vi "Status ProgramSetting.vi"(8 "error in (no error)":errorcluster, 10 "Address (0)":i32, 11 "VISA resource name":refnum<visa-resource-name>) -> (0 "error out":errorcluster, 1 "PRGM Name":string, 2 "PRGM area":i32, 3 "VISA resource name out":refnum<visa-resource-name>, 5 "End condition":T1)   [LabVIEW 2021, in "Environment Chamber.lvlib" / "Climatic Chamber.lvlib"]
doc: "<b>Program assignment monitor</B>\n\nReturns the program area, program pattern name, and end setting of the program operation being executed."
uses:
  Climatic Chamber.lvlib
  Private/Type Defs/Program EndCond Enum.ctl
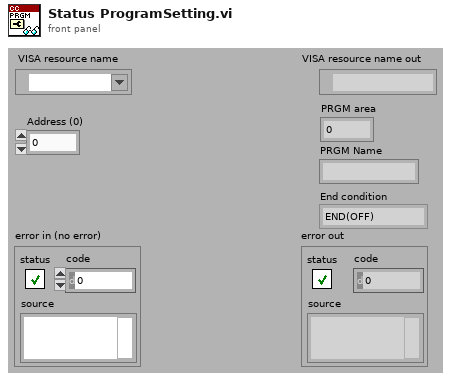
[diagram p1: front panel]
types:
  T1 = typedef "Environment Chamber.lvlib/Climatic Chamber.lvlib/Program EndCond Enum.ctl" = enum16{"END(OFF)", "END(STANDBY)", "END(CONSTANT)", "END(HOLD)", "END(RUN)"}
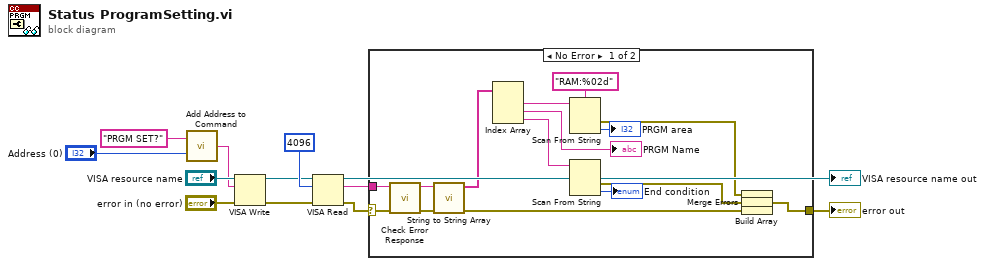
[diagram p0: block diagram]
diagram:
  n1 = call "Add Address to Command.vi"("Address (0)"="Address (0)", "Command"="PRGM SET?") -> ("Command OUT"=w5:string)
  n2 = VISA Write(VISA resource name="VISA resource name", write buffer=w5, error in (no error)="error in (no error)") -> (VISA resource name out=w9:refnum<visa-resource-name>, error out=w8:errorcluster)  [unwired: 1 out]
  n3 = VISA Read(VISA resource name=w9, byte count=u32 4096, error in (no error)=w8) -> (VISA resource name out=→"VISA resource name out":refnum<visa-resource-name>, read buffer=w3:string, error out=w4:errorcluster)  [unwired: 1 out]
  n4 = case shown="No Error" w4 {
    selector: w4 -> [w27 w29]
    tunnel: w3 -> [w28 _]
    tunnel: [w16 w29] -> w2
    frame No Error {
      n5 = call "Check Error Response.vi"("error in (no error)"=w27, "read String"=w28) -> ("error out"=w25:errorcluster, "String out"=w26:string)  [unwired: 7 in, 1 out]
      n6 = call "String to String Array.vi"("error in (no error)"=w25, "String received"=w26) -> ("error out"=w24:errorcluster, "Array Data"=w23:string[])  [unwired: 8 in]
      n7 = Index Array(array=w23) -> (element #1=w22:string, element #2=→"PRGM Name":string, element #3=w18:string)  [unwired: 3 in]
      n8 = Scan From String(format string="RAM:%02d", input string=w22) -> (error out=w15:errorcluster, output 1=→"PRGM area":i32)  [unwired: 3 in, 2 out]
      n9 = Scan From String(input string=w18) -> (error out=w14:errorcluster, output 1=→"End condition":T1)  [unwired: 4 in, 2 out]
      n10 = Build Array(w15, w14, w24) -> (w13:errorcluster[])
      n11 = Merge Errors(w13) -> (w16:errorcluster)
    }
    frame Error {
    }
  }
  "error out" <- w2
